vi "Update Camera Status.vi"(3 "CameraDevRef In":T1, 4 "Enable Vision":bool) -> (0 "CameraDevRef Out":T1)   [LabVIEW 2011]
uses:
  <vilib>/Rock Robotics/WPI/Camera/WPI_CameraDevRef.ctl
  <vilib>/Rock Robotics/WPI/Camera/WPI_CameraSessionID.ctl
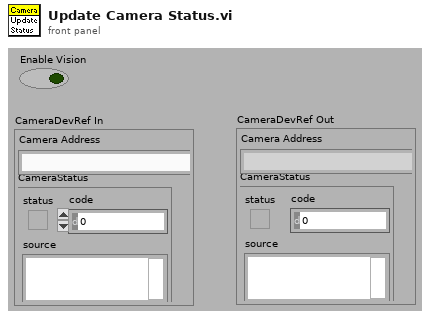
[diagram p1: front panel]
types:
  T1 = typedef "WPI_CameraDevRef.ctl" = cluster{"Camera Address":string, "CameraStatus":errorcluster, "Session ID":T2}
  T2 = typedef "WPI_CameraSessionID.ctl" = i32
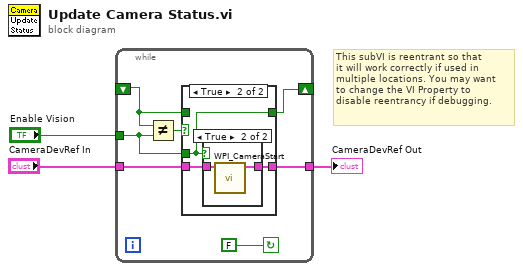
[diagram p0: block diagram]
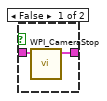
[diagram p3: hidden frame]
diagram:
  # "This subVI is reentrant so that\nit will work correctly if used in\nmultiple locations. You may want\nto change the VI Property to\ndisable reentrancy if debugging."
  n1 = while {
    tunnel: "Enable Vision" -> [w10]
    tunnel: "CameraDevRef In" -> [w8]
    tunnel: [w7] -> w1
    shift-right: [w5] -> _
    shift-left: _ -> [w6]
    stop <- FALSE continue-if-true
    n2 = Not Equal?(x=w6, y=w10) -> (x != y?=w9:bool)
    n3 = case shown="True" w9 {
      tunnel: w8 -> [w12 w15]
      tunnel: [w12 w14] -> w7
      tunnel: [w11 w13] -> w5
      tunnel: w6 -> [w11 _]
      tunnel: w10 -> [_ w13]
      frame False {
      }
      frame True {
        n4 = case shown="True" w13 {
          tunnel: w15 -> [w17 w18]
          tunnel: [w16 w19] -> w14
          frame False {
            n5 = call <vilib>:"WPI_CameraStop.vi"("CameraDevRef"=w17) -> ("CameraDevRef Out"=w16:T1)  [unwired: 1 in, 9 out]
          }
          frame True {
            n6 = call <vilib>:"WPI_CameraStart.vi"("CameraDevRef"=w18) -> ("CameraDevRef Out"=w19:T1)  [unwired: 1 in, 9 out]
          }
        }
      }
    }
  }
  "CameraDevRef Out" <- w1
